vi "Get Instrument Information.vi"(8 "error in (no error)":errorcluster, 10 "Information Tag":string, 11 "Station Config in":refnum<class "Station Config.lvclass">) -> (0 "error out":errorcluster, 3 "Instrument Info":string)   [LabVIEW 2015, in "Station Config.lvlib" / "Station Config.lvclass"]
uses:
  Station Config.lvclass
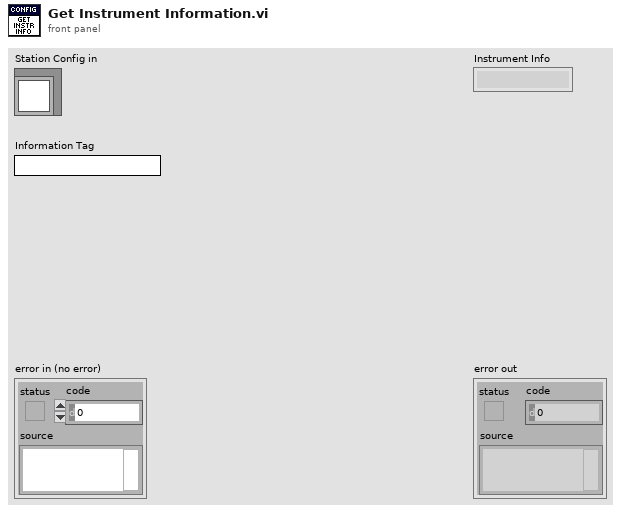
[diagram p1: front panel]
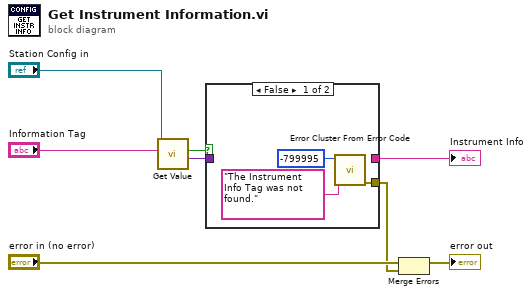
[diagram p0: block diagram]
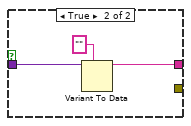
[diagram p2: hidden frame]
diagram:
  n1 = call-dynamic "Get Value.vi"("Key"="Information Tag", "Registry in"="Station Config in") -> ("Value"=w6:variant, "found?"=w7:bool)  [unwired: 6 in, 2 out]
  n2 = case shown="False" w7 {
    tunnel: w6 -> [_ w14]
    tunnel: [_ w13] -> w2
    tunnel: [w11 _] -> w3
    frame False {
      n3 = call <vilib>:"Error Cluster From Error Code.vi"("error message (\"\")"="The Instrument Info Tag was not found." ("error message (\"\")"), "error code (0)"=-799995) -> ("error out"=w11:errorcluster)  [unwired: 7 in]
    }
    frame True {
      n4 = Variant To Data(type="", Variant=w14) -> (data=w13:string)  [unwired: 1 in, 1 out]
    }
  }
  "Instrument Info" <- w2
  n5 = Merge Errors("error in (no error)", w3) -> (→"error out":errorcluster)
